vi "ZUP Initialize COM.vi"(8 "error in (no error)":errorcluster, 11 "VISA resource name":refnum<visa-resource-name>) -> (0 "error out":errorcluster, 3 "VISA OUT":refnum<visa-resource-name>)   [LabVIEW 2018]
doc: "This VI uses the serial port specified in \"VISA name\" to send the \"Address\" command to the Genesys power supply. You must run this VI before using any of the instrument driver VIs for this instrument.\n\nYou can optionally reset the instrument by setting the front panel reset control. \nYou can optionally read the instrument identity string and verify ithe instrument can be used with this driver.\n\nThe Timeout is the number of seconds allowed for instrument to respond. The default is 3 seconds."
uses:
  <vilib>/Instr/_visa.llb/VISA Configure Serial Port (Instr).vi
panel:
  # "Lambda ZUP \n Serial Port\n  DC Power Supplies"
  # "Initialize Instrument\nOpen VISA Port"
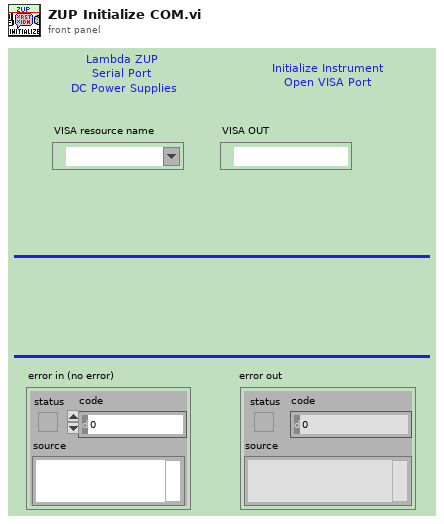
[diagram p1: front panel]
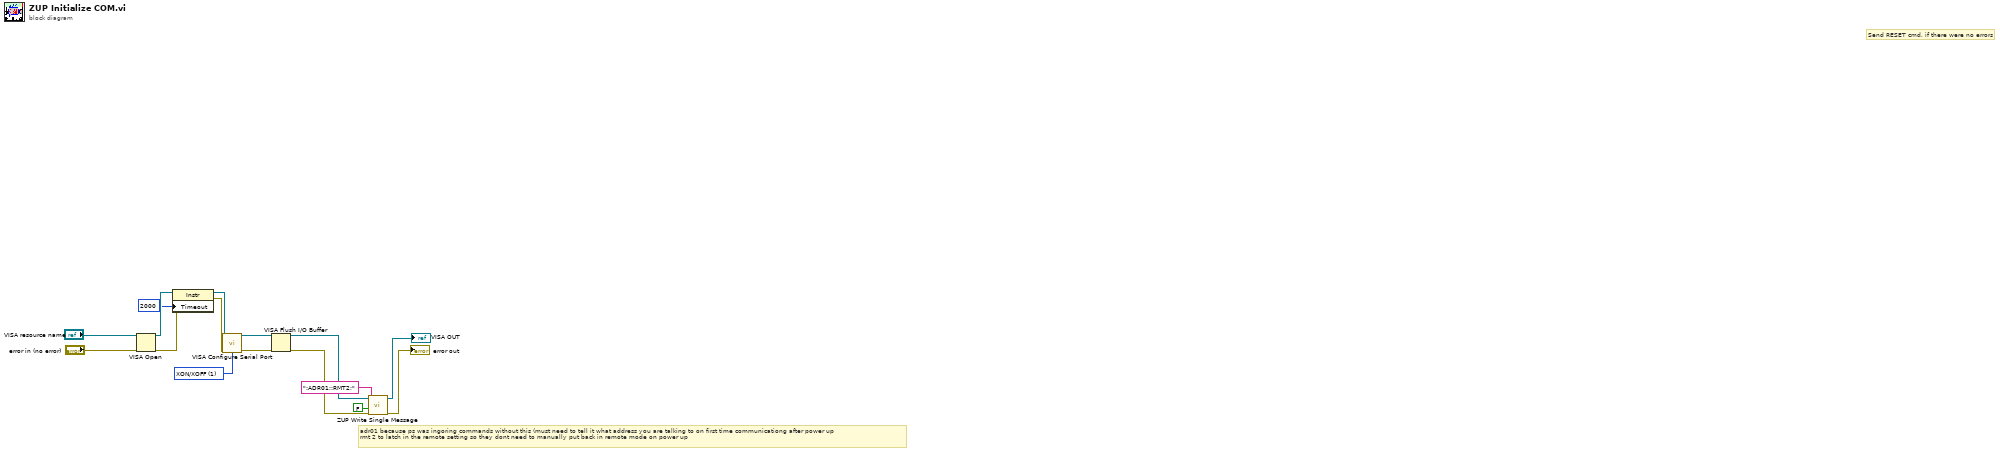
[diagram p0: block diagram]
diagram:
  w13 = u16 1 items=["None", "XON/XOFF", "RTS/CTS", "XON/XOFF & RTS/CTS", "DTR/DSR", "XON/XOFF & DTR/DSR"] ("flow control (0:none)")
  # "adr01 because ps was ingoring commands without this (must need to tell it what address you are talking to on first time communicationg after power up\nrmt 2 to latch in the remote setting so they dont need to manually put back in remote mode on power up"
  # "Send RESET cmd, if there were no errors"
  n1 = VISA Open(error in (no error)="error in (no error)", VISA resource name="VISA resource name") -> (VISA resource name=w12:refnum<visa-resource-name>, error out=w9:errorcluster)  [unwired: 3 in]
  n2 = property class="Instr"(reference=w12, error in=w9, "Timeout"=u32 2000 ("General Settings:Timeout Value")) -> (reference out=w11:refnum<visa-resource-name>, error out=w8:errorcluster)
  n3 = call-poly "VISA Configure Serial Port"("VISA resource name"=w11, "error in (no error)"=w8, "flow control (0:none)"=w13) -> ("VISA resource name out"=w14:refnum<visa-resource-name>, "error out"=w15:errorcluster)  [unwired: 11 in]
  n4 = VISA Flush I/O Buffer(VISA resource name=w14, error in (no error)=w15) -> (VISA resource name out=w5:refnum<visa-resource-name>, error out=w4:errorcluster)  [unwired: 1 in]
  n5 = call "ZUP Write Single Message.vi"("error in (no error)"=w4, "Read Response"=FALSE, "Command Out"=":ADR01;:RMT2;", "VISA resource name"=w5) -> ("error out"=→"error out":errorcluster, "VISA OUT"=→"VISA OUT":refnum<visa-resource-name>)  [unwired: 4 in, 2 out]
